vi "WriteToFile-2D.vi"(0 "Refnum in":refnum<k34>, 1 "Group Name":string, 3 "Channel Names":string[](array[string]), 5 "rt fifo":refnum<k33>, 7 "File array":dbl[][](array[numeric]), 9 "Write?":bool, 11 "error in (no error)":errorcluster, 12 "index":i32) -> (4 "Refnum out":refnum<k34>, 8 "File array 2":dbl[][](array[numeric]), 10 "Writing to file":bool, 15 "error out":errorcluster)   [LabVIEW 2018]
uses:
  d1328624-c948-4157-a192-2ea999cd4fd4.vi
  <vilib>/Array/Sort 2D Array - Pop Stack.vi
  <vilib>/Array/Sort 2D Array - Push Stack.vi
  d1328624-c948-4157-a192-2ea999cd4fd4.vi/6c9825cd-1e20-4146-b36d-d941b11e5da5.vi
  d1328624-c948-4157-a192-2ea999cd4fd4.vi/d77664fb-eb25-43ad-903d-0cc263163e4c.vi
panel:
  out "output array":dbl[][](array[numeric])
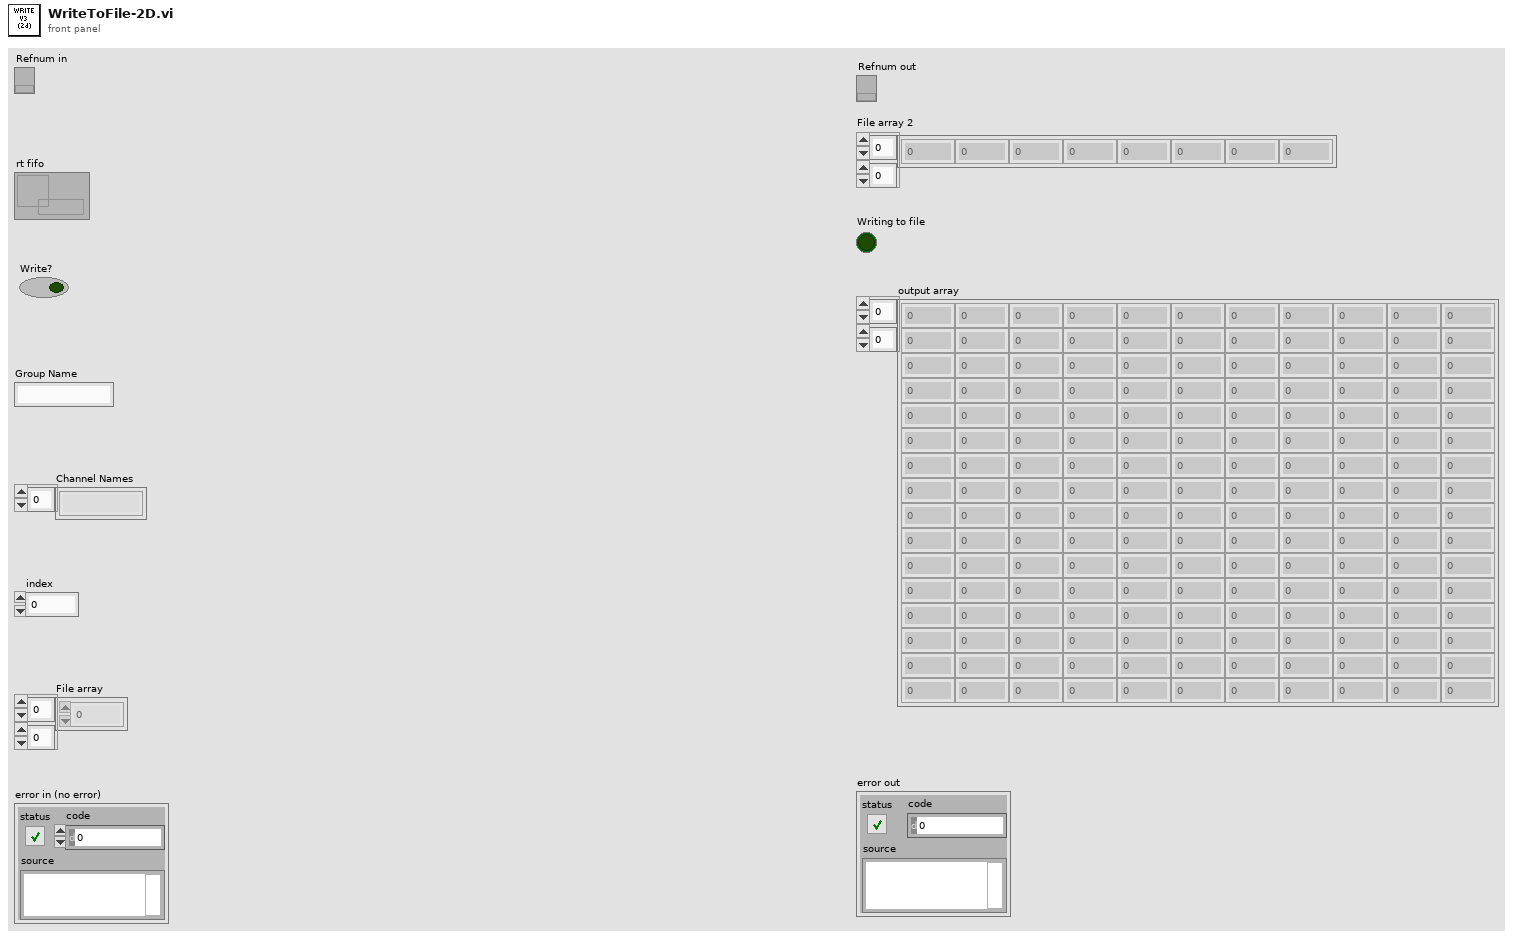
[diagram p1: front panel]
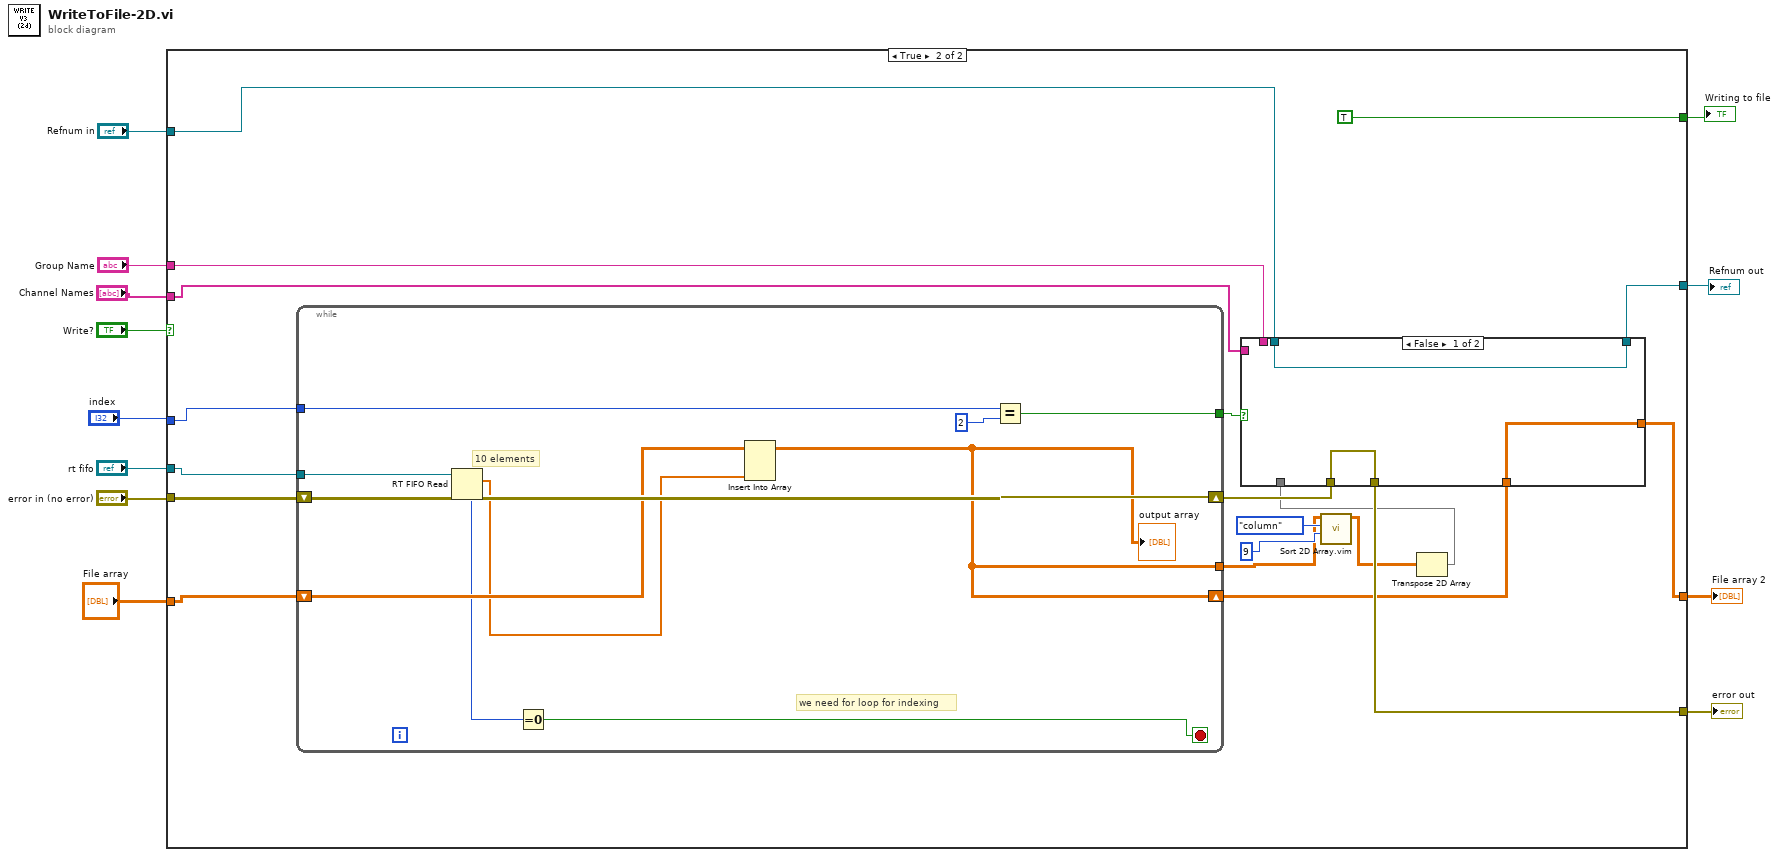
[diagram p0: block diagram]
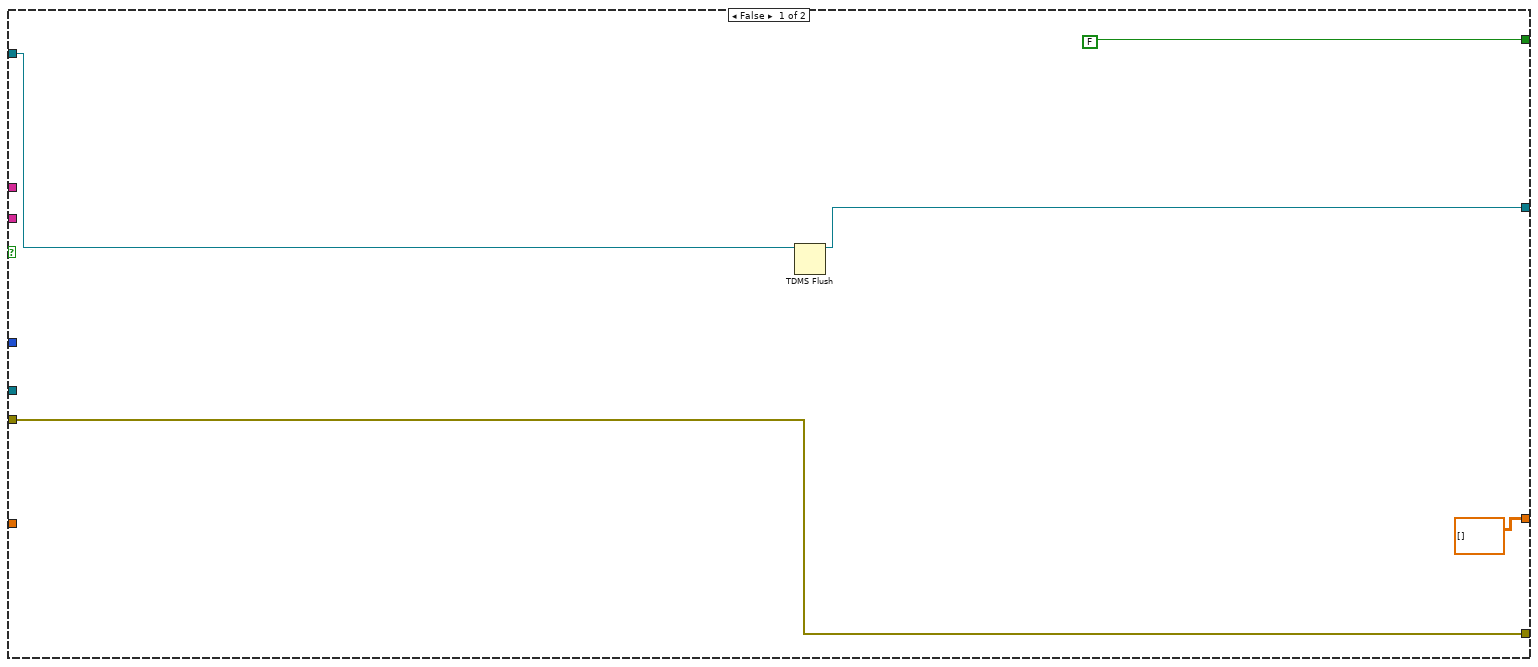
[diagram p2: hidden frame]
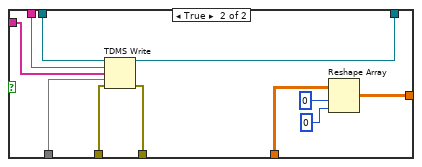
[diagram p3: hidden frame]
diagram:
  n1 = case shown="True" "Write?" {
    tunnel: "Refnum in" -> [w15 w31]
    tunnel: [w13 w27] -> w8
    tunnel: [w16 w35] -> w9
    tunnel: "Channel Names" -> [_ w32]
    tunnel: "Group Name" -> [_ w33]
    tunnel: [FALSE ("Writing to file") TRUE ("Writing to file")] -> w6
    tunnel: "rt fifo" -> [_ w30]
    tunnel: "error in (no error)" -> [w16 w34]
    tunnel: [dbl[][] [] ("File array") w18] -> w3
    tunnel: "index" -> [_ w26]
    tunnel: "File array" -> [_ w20]
    frame False {
      n2 = TDMS Flush(7:w15) -> (3:w13:refnum<k34>)  [unwired: 1 in, 1 out]
    }
    frame True {
      n3 = while {
        tunnel: w30 -> [w61]
        shift-right: [w59] -> w29
        shift-left: w34 -> [w60]
        tunnel: [w57] -> w28
        tunnel: w26 -> [w52]
        tunnel: [w51] -> w21
        shift-right: [w51] -> w19
        shift-left: w20 -> [w55]
        stop <- w56 stop-if-true
        # "we need for loop for indexing"
        # "10 elements"
        n4 = RT FIFO Read(0:w61, 3:w60) -> (7:w53:u32, 9:w54:dbl[], 11:w59:errorcluster)  [unwired: 2 in, 2 out]
        n5 = Equal To 0?(x=w53) -> (x = 0?=w56:bool)
        n6 = Insert Into Array(array=w55, new element=w54) -> (w51:dbl[][])  [unwired: 2 in]
        "output array" <- w51
        n7 = Equal?(x=w52, y=2) -> (x = y?=w57:bool)
      }
      n8 = call "Sort 2D Array.vim"("index"=9, "dimension to index (column)"=enum16{"column", "row"}."column", "2D array"=w21) -> ("sorted 2D array"=w23:dbl[][])  [unwired: 7 in, 1 out]
      n9 = Transpose 2D Array(2D array=w23) -> (transposed array=w22:dbl[][])
      n10 = case shown="False" w28 {
        tunnel: w32 -> [_ w50]
        tunnel: w33 -> [_ w49]
        tunnel: w31 -> [w39 w48]
        tunnel: [w38 w47] -> w35
        tunnel: [w39 w46] -> w27
        tunnel: w29 -> [w38 w45]
        tunnel: w22 -> [_ w44]
        tunnel: w19 -> [w37 w43]
        tunnel: [w37 w40] -> w18
        frame False {
        }
        frame True {
          n11 = TDMS Write(0:w48, 5:w49, 7:w50, 9:w44, 11:w45) -> (4:w46:refnum<k34>, 15:w47:errorcluster)  [unwired: 1 in, 2 out]
          n12 = Reshape Array(w43, 0 ("dimension size"), 0 ("dimension size")) -> (w40:dbl[][])
        }
      }
    }
  }
  "error out" <- w9
  "Refnum out" <- w8
  "Writing to file" <- w6
  "File array 2" <- w3
